vi "_Parse SEM Margin Result.vi"(8 "error in (no error)":errorcluster, 10 "Input String":string, 11 "VISA resource name":refnum<visa-resource-name>) -> (0 "error out":errorcluster, 1 "Results":cluster{"Margin X":dbl, "Margin Y":dbl}[](array[cluster]), 2 "Reliability":i32, 3 "VISA resource name out":refnum<visa-resource-name>, 5 "Out Of Tolerance":dbl format="%^.3e")   [LabVIEW 2015, in "Rohde&Schwarz CMXP NR FR2 Measurement.lvlib"]
uses:
  <instrlib>/Rohde&Schwarz CMXP NR FR2 Measurement/Rohde&Schwarz CMXP NR FR2 Measurement.lvlib
  <instrlib>/Rohde&Schwarz CMXP NR FR2 Measurement/Private/rsidr_core.llb/rsidr_core.lvlib
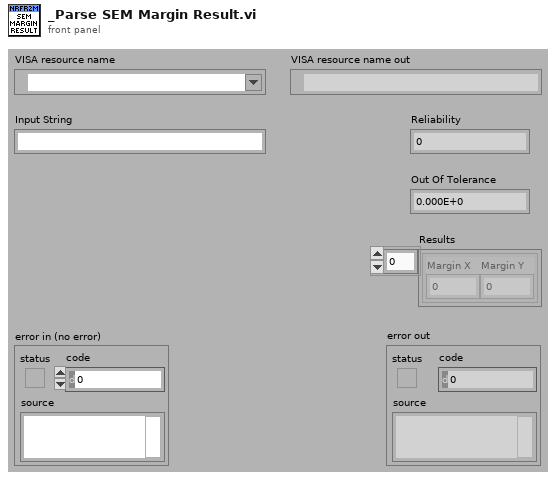
[diagram p1: front panel]
types:
  T1 = cluster{"double array out[0]":dbl, "double array out[1]":dbl}
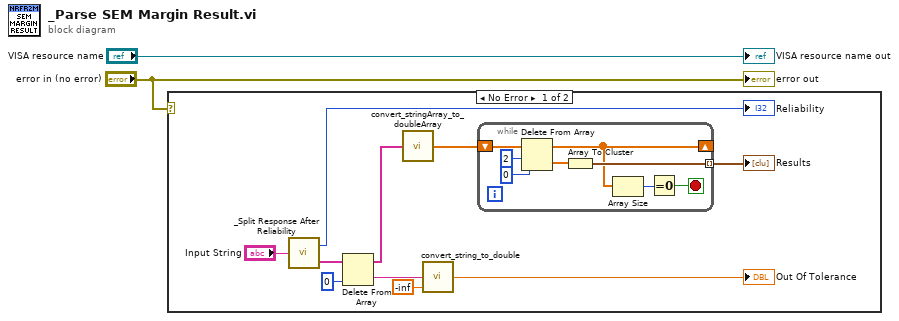
[diagram p0: block diagram]
diagram:
  n1 = case shown="No Error" "error in (no error)" {
    frame No Error {
      n2 = call <instrlib>:"_Split Response After Reliability.vi"("Input String"="Input String") -> ("Response out"=w8:string[], "Reliability out"=→"Reliability":i32)
      n3 = Delete From Array(array=w8, index=0) -> (deleted portion=w6:string, array with subset deleted=w5:string[])  [unwired: 1 in]
      n4 = call <instrlib>:"convert_stringArray_to_doubleArray.vi"("string array in"=w5) -> ("double array out"=w3:dbl[])  [unwired: 4 in]
      n5 = call <instrlib>:"convert_string_to_double.vi"("default (0)"=-inf, "String in"=w6) -> ("double value out"=→"Out Of Tolerance":dbl)  [unwired: 3 in]
      n6 = while {
        shift-right: [w15] -> _
        shift-left: w3 -> [w20]
        tunnel: [w16] -> w4 mode=indexing
        stop <- w13 stop-if-true
        n7 = Delete From Array(array=w20, length=2, index=0) -> (deleted portion=w17:dbl[], array with subset deleted=w15:dbl[])
        n8 = Array To Cluster(array=w17) -> (cluster=w16:T1)
        n9 = Array Size(array=w15) -> (size(s)=w14:i32)
        n10 = Equal To 0?(x=w14) -> (x = 0?=w13:bool)
      }
      "Results" <- w4
    }
    frame Error {
    }
  }
  "error out" <- "error in (no error)"
  "VISA resource name out" <- "VISA resource name"
